vi "Trigger Freigabe.vi"(6 "Aktion":T1, 8 "error in (no error)":errorcluster caption="Fehler (Eingang, kein Fehler)") -> (0 "error out":errorcluster caption="Fehler (Ausgang)", 3 "Freigabe":bool)   [LabVIEW 2015, in "Schedule Modul.lvlib"]
uses:
  Schedule Modul.lvlib
  Aktion Trigger Freigabe.ctl
  Aktion FGV Schedule Daten.ctl
  Funktionstasten/Funktionstasten-Aktion.ctl
  Funktionstasten/Zustaende.ctl
  Funktionstasten/Funktionstasten.lvlib
panel:
  out "Fehler steht an":bool
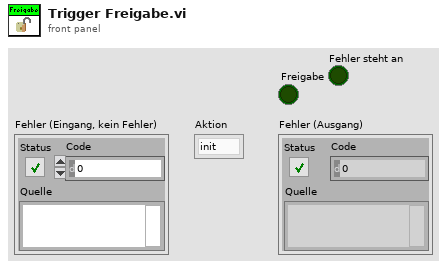
[diagram p1: front panel]
types:
  T1 = typedef "Schedule Modul.lvlib/Aktion Trigger Freigabe.ctl" = enum16{"init", "lesen", "prüfen", "löschen"}
  T2 = typedef "Funktionstasten.lvlib/Zustaende.ctl" = enum16{"Standby", "Pause", "Eco", "Messen", "Kalibrieren", "Spülen Filter", "Spülen Leitung", "0-Gas", "Cal-Gas", "CG zu PNS", "-------------", "Init 1", "Init 2", "Init 3", "Init 4", "Messen vorbereiten", "Messen durchführen", "Exit"}
  T3 = typedef "Funktionstasten.lvlib/Funktionstasten-Aktion.ctl" = enum16{"Initialisieren", "Zustand setzen", "Taste gedrückt", "Fehler speichern", "Lesen", "Manuell", "Remote", "Bitparallel", "Samplepoint", "Zeit Prüfen", "reset Umschalten"}
  T4 = typedef "Schedule Modul.lvlib/Aktion FGV Schedule Daten.ctl" = enum16{"lesen", "laden", "speichern", "schreiben"}
  T5 = typedef "Schedule Modul.lvlib/Aktive Wochentage.ctl" = cluster{"Montag":bool, "Dienstag":bool, "Mittwoch":bool, "Donnerstag":bool, "Freitag":bool, "Samstag":bool, "Sonntag":bool}
  T6 = typedef "Schedule Modul.lvlib/Zeitstempel.ctl" = cluster{"Montag":T7, "Dienstag":T7, "Mittwoch":T7, "Donnerstag":T7, "Freitag":T7, "Samstag":T7, "Sonntag":T7}
  T7 = typedef "Schedule Modul.lvlib/Zeitstempel-Bedienelement.ctl" = timestamp
  T8 = typedef "Schedule Modul.lvlib/Planer Status.ctl" = u16
  T9 = cluster{"second":i32, "minute":i32, "hour":i32, "day of month":i32, "month":i32, "year":i32, "day of week":i32, "day of year":i32, "is DST":i32}
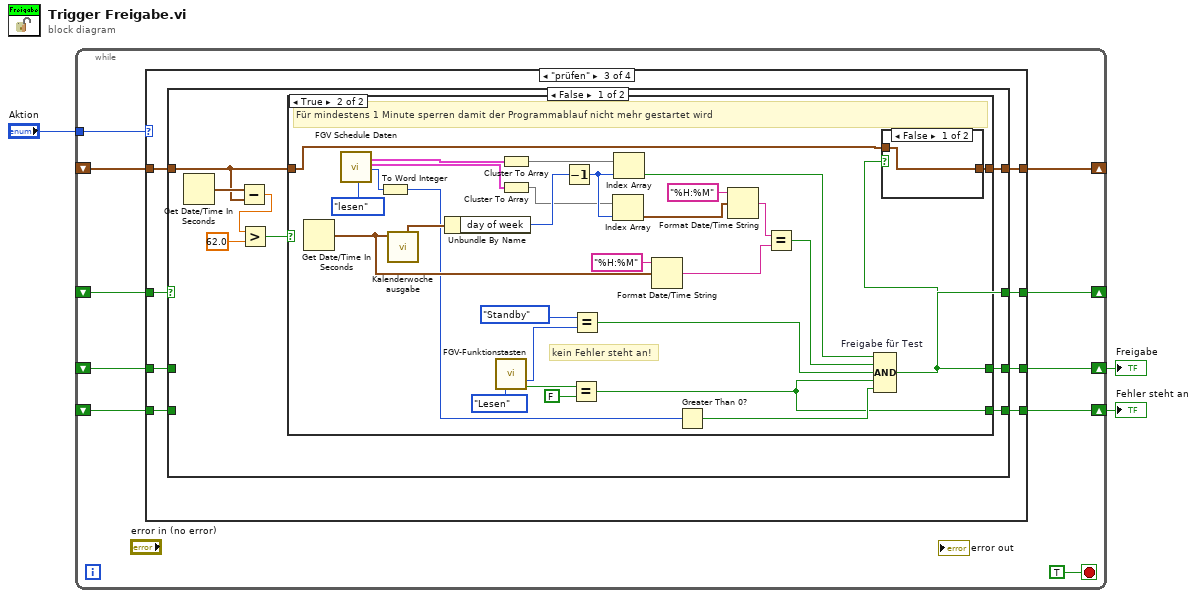
[diagram p0: block diagram]
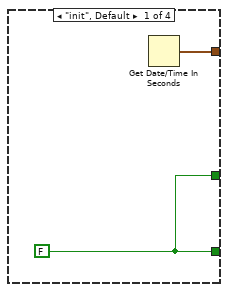
[diagram p2: hidden frame]
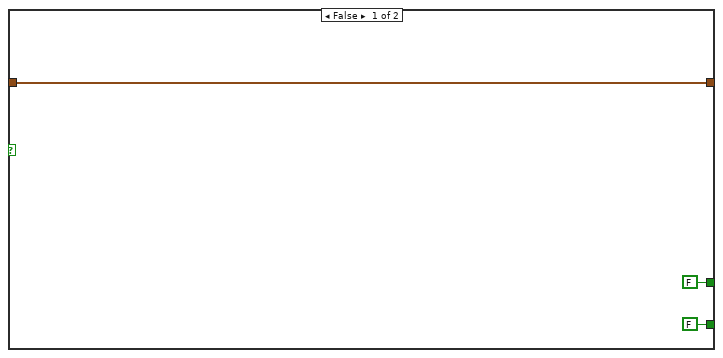
[diagram p4: hidden frame]
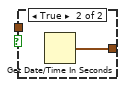
[diagram p5: hidden frame]
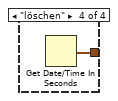
[diagram p7: hidden frame]
diagram:
  n1 = while {
    shift-right: [w12] -> w2
    shift-left: _ -> [w11]
    tunnel: "Aktion" -> [w10]
    shift-right: [w9] -> _
    shift-left: _ -> [w8]
    shift-right: [w7] -> w1
    shift-left: _ -> [w6]
    shift-right: [w5] -> _
    shift-left: _ -> [w4]
    stop <- TRUE stop-if-true
    n2 = case shown="\"prüfen\"" w10 {
      tunnel: [w15 w17 w26 _] -> w12
      tunnel: w11 -> [_ w17 w24 _]
      tunnel: [w15 w18 w23 _] -> w9
      tunnel: w8 -> [_ w18 w25 _]
      tunnel: [_ _ w22 _] -> w7
      tunnel: w6 -> [_ _ w21 _]
      tunnel: [w14 w16 w20 w73] -> w5
      tunnel: w4 -> [_ w16 w19 _]
      frame "init", Default {
        w15 = FALSE
        n3 = Get Date/Time In Seconds() -> (seconds since 1Jan1904=w14:timestamp)
      }
      frame "lesen" {
      }
      frame "prüfen" {
        n4 = case shown="False" w25 {
          selector: w25 -> [_ w71]
          tunnel: [w33 w72] -> w26
          tunnel: w24 -> [_ w72]
          tunnel: [w33 w71] -> w23
          tunnel: [w34 w70] -> w22
          tunnel: w21 -> [_ w70]
          tunnel: [w32 w69] -> w20
          tunnel: w19 -> [w27 w69]
          frame False {
            n5 = Get Date/Time In Seconds() -> (seconds since 1Jan1904=w28:timestamp)
            n6 = Subtract(x=w28, y=w27) -> (x-y=w31:dbl)
            n7 = Greater?(x=w31, y=62.0) -> (0:w29:bool)
            n8 = case shown="True" w29 {
              tunnel: [FALSE w43] -> w34
              tunnel: [FALSE w42] -> w33
              tunnel: [w37 w41] -> w32
              tunnel: w27 -> [w37 w40]
              frame False {
              }
              frame True {
                # "kein Fehler steht an!"
                # "Für mindestens 1 Minute sperren damit der Programmablauf nicht mehr gestartet wird"
                n9 = Get Date/Time In Seconds() -> (seconds since 1Jan1904=w58:timestamp)
                n10 = call "FGV Schedule Daten.vi"("Aktion"=Aktion_FGV_Schedule_Daten."lesen") -> ("Aktive Wochentage"=w64:T5, "Zeiten"=w61:T6, "Planer Status"=w39:T8)  [unwired: 13 in, 3 out]
                n11 = To Word Integer(number=w39) -> (16bit integer=w45:i16)
                n12 = call "Kalenderwoche ausgabe.vi"("Date (now)"=w58) -> ("Date ISO"=w65:T9)  [unwired: 4 in, 6 out]
                n13 = Unbundle By Name(w65) -> ("day of week"=w62:i32)
                n14 = call "FGV-Funktionstasten.vi"("Aktion"=Funktionstasten-Aktion."Lesen") -> ("ausgewählte Funktion"=w50:T2, "Fehler steht an"=w51:bool)  [unwired: 7 in, 6 out]
                n15 = Cluster To Array(cluster=w64) -> (array=w63:bool[])
                n16 = Cluster To Array(cluster=w61) -> (array=w59:T7[])
                n17 = Decrement(x=w62) -> (x-1=w60:i32)
                n18 = Equal?(x=w51, y=FALSE) -> (x = y?=w43:bool)
                n19 = Equal?(x=Zustaende."Standby", y=w50) -> (x = y?=w46:bool)
                n20 = Index Array(array=w59, index=w60) -> (element=w55:T7)
                n21 = Index Array(array=w63, index=w60) -> (element=w48:bool)
                n22 = Format Date/Time String(time format string (%c)="%H:%M" ("Zeitformatierungs-String (%c)"), seconds (now)=w58) -> (date/time string=w53:string)  [unwired: 1 in]
                n23 = Greater Than 0?(x=w45) -> (x > 0?=w44:bool)
                n24 = Format Date/Time String(time format string (%c)="%H:%M" ("Zeitformatierungs-String (%c)"), seconds (now)=w55) -> (date/time string=w54:string)  [unwired: 1 in]
                n25 = Equal?(x=w54, y=w53) -> (x = y?=w47:bool)
                n26 = Compound Arithmetic op=AND "Freigabe für Test"(w48, w47, w46, w43, w44) -> (w42:bool)
                n27 = case shown="False" w42 {
                  tunnel: [w67 w68] -> w41
                  tunnel: w40 -> [w67 _]
                  frame False {
                  }
                  frame True {
                    n28 = Get Date/Time In Seconds() -> (seconds since 1Jan1904=w68:timestamp)
                  }
                }
              }
            }
          }
          frame True {
          }
        }
      }
      frame "löschen" {
        n29 = Get Date/Time In Seconds() -> (seconds since 1Jan1904=w73:timestamp)
      }
    }
  }
  "Freigabe" <- w2
  "Fehler steht an" <- w1
